vi "index array (dbl with idx).vi"(4 "Indices":i32[](array[numeric]), 5 "array":dbl[](array[numeric])) -> (1 "indexed array":dbl[](array[numeric]))   [LabVIEW 2012, in "common.lvlib"]
uses:
  common.lvlib
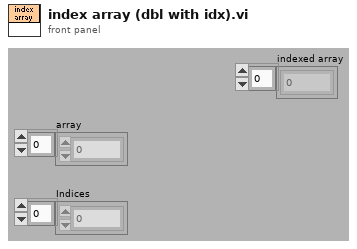
[diagram p1: front panel]
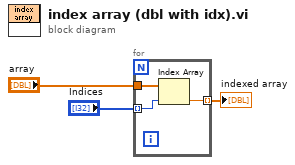
[diagram p0: block diagram]
diagram:
  n1 = for {
    tunnel: "Indices" -> [w5] mode=indexing
    tunnel: "array" -> [w6]
    tunnel: [w4] -> w1 mode=indexing
    n2 = Index Array(array=w6, index=w5) -> (element=w4:dbl)
  }
  "indexed array" <- w1
